vi "Set 2D Picture.vi"(8 "error in (no error)":errorcluster, 10 "picture":picture) -> (0 "error out":errorcluster, 1 "Valid":bool, 3 "Grassfire out":refnum<class "Grassfire.lvclass">)   [LabVIEW 2019, in "Grassfire.lvclass"]
uses:
  Grassfire.lvclass
  Grassfire.lvclass/Grassfire.ctl
  Node/Node.lvclass
  Address/Address.lvclass
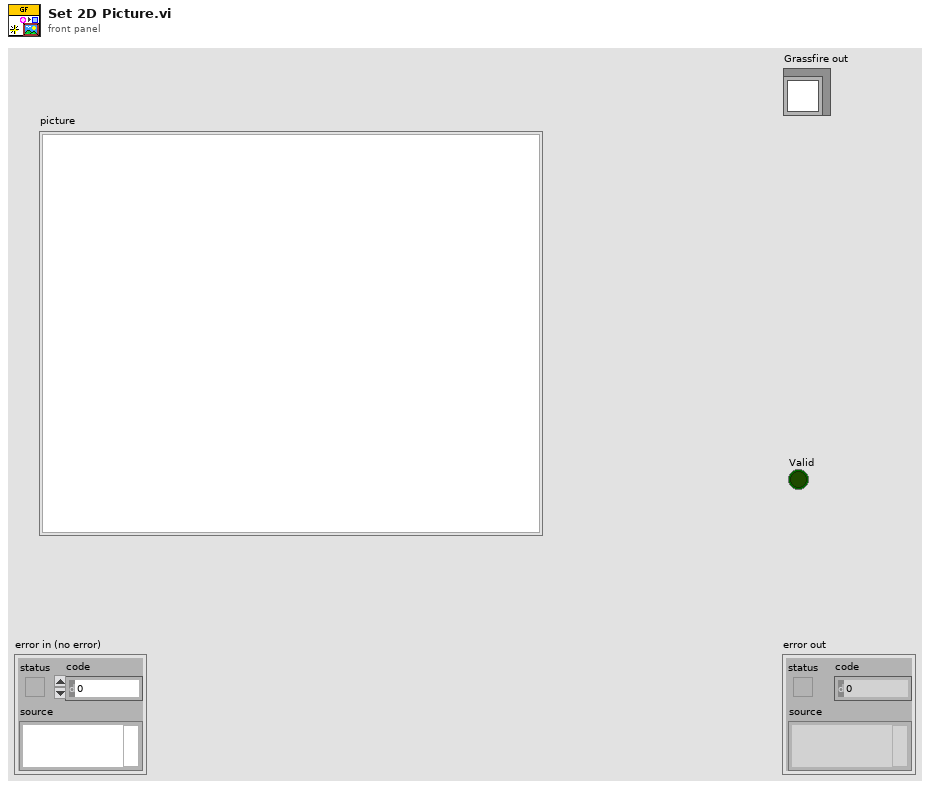
[diagram p1: front panel]
types:
  T1 = typedef "imagedata.ctl" = cluster{"image type":i32, "image depth":i32, "image":u8[], "mask":u8[], "colors":u32[], "Rectangle":cluster{"left":i16, "top":i16, "right":i16, "bottom":i16}}
  T2 = cluster{"Empty":refnum<class "Node.lvclass">, "Blocked":refnum<class "Node.lvclass">, "Start":refnum<class "Node.lvclass">, "End":refnum<class "Node.lvclass">, "Path":refnum<class "Node.lvclass">}
  T3 = map{refnum<class "Address.lvclass">, refnum<class "Node.lvclass">}
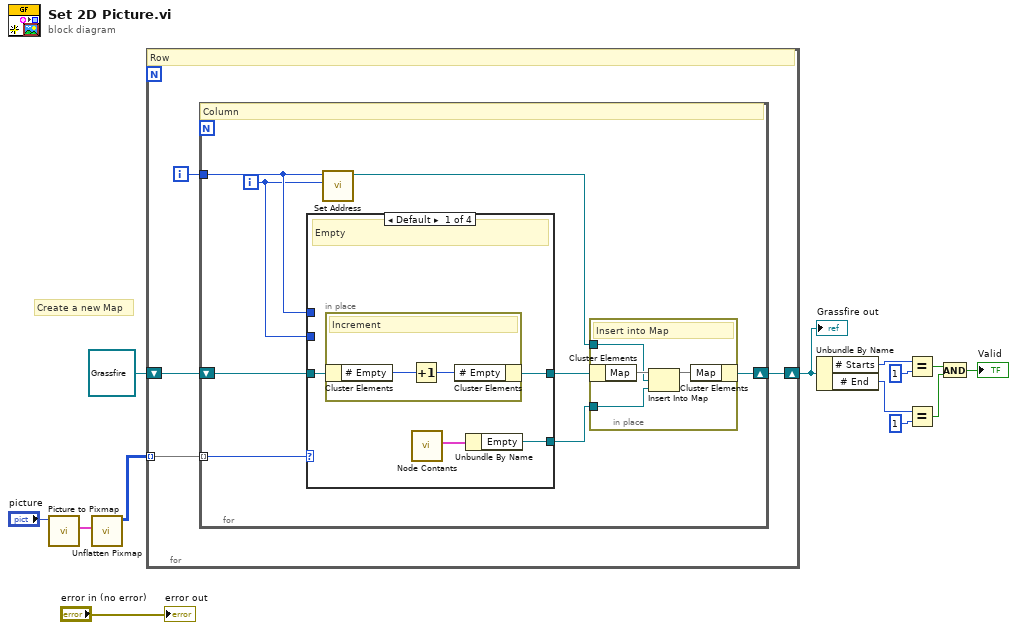
[diagram p0: block diagram]
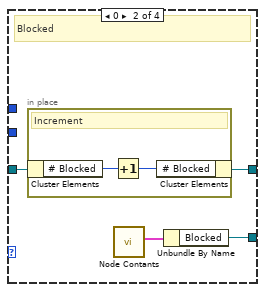
[diagram p2: hidden frame]
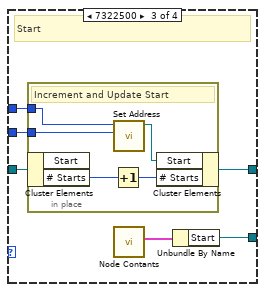
[diagram p3: hidden frame]
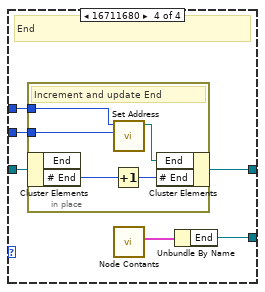
[diagram p4: hidden frame]
diagram:
  # "Create a new Map"
  n1 = call <vilib>:"Picture to Pixmap.vi"("picture"="picture") -> ("image data"=w3:T1)  [unwired: 9 in, 1 out]
  n2 = call <vilib>:"Unflatten Pixmap.vi"("image data"=w3) -> ("24-bit pixmap"=w2:u32[][])  [unwired: 4 in, 6 out]
  n3 = for {
    tunnel: w2 -> [w17] mode=indexing
    shift-right: [w14] -> w4
    shift-left: refnum<class "Grassfire.lvclass"> refnum ("Grassfire out") -> [w15]
    i -> [w16]
    # "Row"
    n4 = for {
      tunnel: w17 -> [w18] mode=indexing
      tunnel: w16 -> [w25]
      shift-right: [w21] -> w14
      shift-left: w15 -> [w23]
      i -> [w24]
      # "Column"
      n5 = case shown="Default" w18 {
        tunnel: w23 -> [w33 w39 w47 w58]
        tunnel: [w32 w38 w46 w57] -> w22
        tunnel: w25 -> [_ _ w45 w56]
        tunnel: w24 -> [_ _ w44 w55]
        tunnel: [w30 w36 w42 w53] -> w19
        frame Default {
          # "Empty"
          n6 = in-place {
            # "Increment"
            n7 = in-place-cluster #1(w33) -> ("# Empty"=w35:i32)
            n8 = Increment(x=w35) -> (x+1=w34:i32)
            n9 = in-place-cluster #1("# Empty"=w34) -> (w32:refnum<class "Grassfire.lvclass">)
          }
          n10 = call "Node Contants.vi"() -> ("Constants"=w31:T2)  [unwired: 10 in, 1 out]
          n11 = Unbundle By Name(w31) -> ("Empty"=w30:refnum<class "Node.lvclass">)
        }
        frame 0 {
          # "Blocked"
          n12 = in-place {
            # "Increment"
            n13 = in-place-cluster #2(w39) -> ("# Blocked"=w41:i32)
            n14 = Increment(x=w41) -> (x+1=w40:i32)
            n15 = in-place-cluster #2("# Blocked"=w40) -> (w38:refnum<class "Grassfire.lvclass">)
          }
          n16 = call "Node Contants.vi"() -> ("Constants"=w37:T2)  [unwired: 10 in, 1 out]
          n17 = Unbundle By Name(w37) -> ("Blocked"=w36:refnum<class "Node.lvclass">)
        }
        frame 7322500 {
          # "Start"
          n18 = in-place {
            in-place-border: w45 -> [w50]
            in-place-border: w44 -> [w49]
            # "Increment and Update Start"
            n19 = in-place-cluster #3(w47) -> ("# Starts"=w52:i32)  [unwired: 1 out]
            n20 = Increment(x=w52) -> (x+1=w51:i32)
            n21 = call "Set Address.vi"("Column"=w49, "Row"=w50) -> ("2D Array Index"=w48:refnum<class "Address.lvclass">)  [unwired: 9 in]
            n22 = in-place-cluster #3("Start"=w48, "# Starts"=w51) -> (w46:refnum<class "Grassfire.lvclass">)
          }
          n23 = call "Node Contants.vi"() -> ("Constants"=w43:T2)  [unwired: 10 in, 1 out]
          n24 = Unbundle By Name(w43) -> ("Start"=w42:refnum<class "Node.lvclass">)
        }
        frame 16711680 {
          # "End"
          n25 = in-place {
            in-place-border: w56 -> [w61]
            in-place-border: w55 -> [w60]
            # "Increment and update End"
            n26 = in-place-cluster #4(w58) -> ("# End"=w63:i32)  [unwired: 1 out]
            n27 = Increment(x=w63) -> (x+1=w62:i32)
            n28 = call "Set Address.vi"("Column"=w60, "Row"=w61) -> ("2D Array Index"=w59:refnum<class "Address.lvclass">)  [unwired: 9 in]
            n29 = in-place-cluster #4("End"=w59, "# End"=w62) -> (w57:refnum<class "Grassfire.lvclass">)
          }
          n30 = call "Node Contants.vi"() -> ("Constants"=w54:T2)  [unwired: 10 in, 1 out]
          n31 = Unbundle By Name(w54) -> ("End"=w53:refnum<class "Node.lvclass">)
        }
      }
      n32 = call "Set Address.vi"("Column"=w24, "Row"=w25) -> ("2D Array Index"=w20:refnum<class "Address.lvclass">)  [unwired: 9 in]
      n33 = in-place {
        in-place-border: w20 -> [w27]
        in-place-border: w19 -> [w26]
        # "Insert into Map"
        n34 = in-place-cluster #5(w22) -> ("Map"=w29:T3)
        n35 = Insert Into Map(map in=w29, key=w27, value=w26) -> (map out=w28:T3)  [unwired: 2 out]
        n36 = in-place-cluster #5("Map"=w28) -> (w21:refnum<class "Grassfire.lvclass">)
      }
    }
  }
  "Grassfire out" <- w4
  n37 = Unbundle By Name(w4) -> ("# Starts"=w7:i32, "# End"=w6:i32)
  n38 = Equal?(x=w7, y=1) -> (x = y?=w10:bool)
  n39 = Equal?(x=w6, y=1) -> (x = y?=w8:bool)
  n40 = And(x=w10, y=w8) -> (x .and. y?=→"Valid":bool)
  "error out" <- "error in (no error)"
